vi "SPCStatus_6629.vi"(1 "Set/Get":bool, 2 "Status (input)":enum16{"offline", "online", "busy"}(ring)) -> (0 "Status (output)":enum16{"offline", "online", "busy"}(ring))   [LabVIEW 2009]
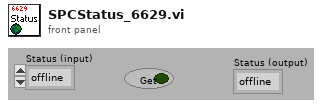
[diagram p1: front panel]
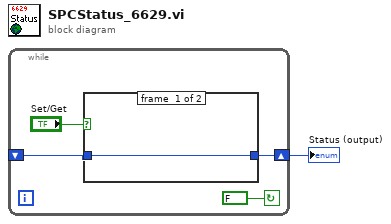
[diagram p0: block diagram]
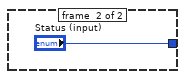
[diagram p2: hidden frame]
diagram:
  n1 = while {
    shift-right: [w3] -> w1
    shift-left: _ -> [w2]
    stop <- FALSE continue-if-true
    n2 = case shown="True" "Set/Get" {
      tunnel: [w6 "Status (input)"] -> w3
      tunnel: w2 -> [w6 _]
      frame #0 {
      }
      frame #1 {
      }
    }
  }
  "Status (output)" <- w1
